vi "RS232_命令(2條直線要寫入雷射的)_VI.vi"(0 "量測值Array(X)":dbl, 1 "量測值Array(Y)":dbl, 2 "功率右":u8=70 max=80, 3 "掃描速率(刀速)右":u16=220 max=2000 format="%0.0f", 5 "error in (no error)":errorcluster, 6 "線段":enum16{"左邊線段", "右邊線段"}(ring), 7 "功率左":u8=70 max=80, 8 "角度(左)":dbl min=0.0 max=360.0, 9 "掃描速率(刀速) 左":u16=220 max=2000 format="%0.0f", 10 "角度(右)":dbl min=0.0 max=360.0, 11 "線段長度左":dbl min=0.0 max=999.0, 13 "線段長度右":dbl) -> (14 "命令字串":string, 19 "error out":errorcluster)   [LabVIEW 2015]
panel:
  out "角度":dbl
  out "X座標":dbl
  out "角度 2":string="-20.000"
  out "X座標 2":string="-20.000"
  out "命令Array":string[](array[string])
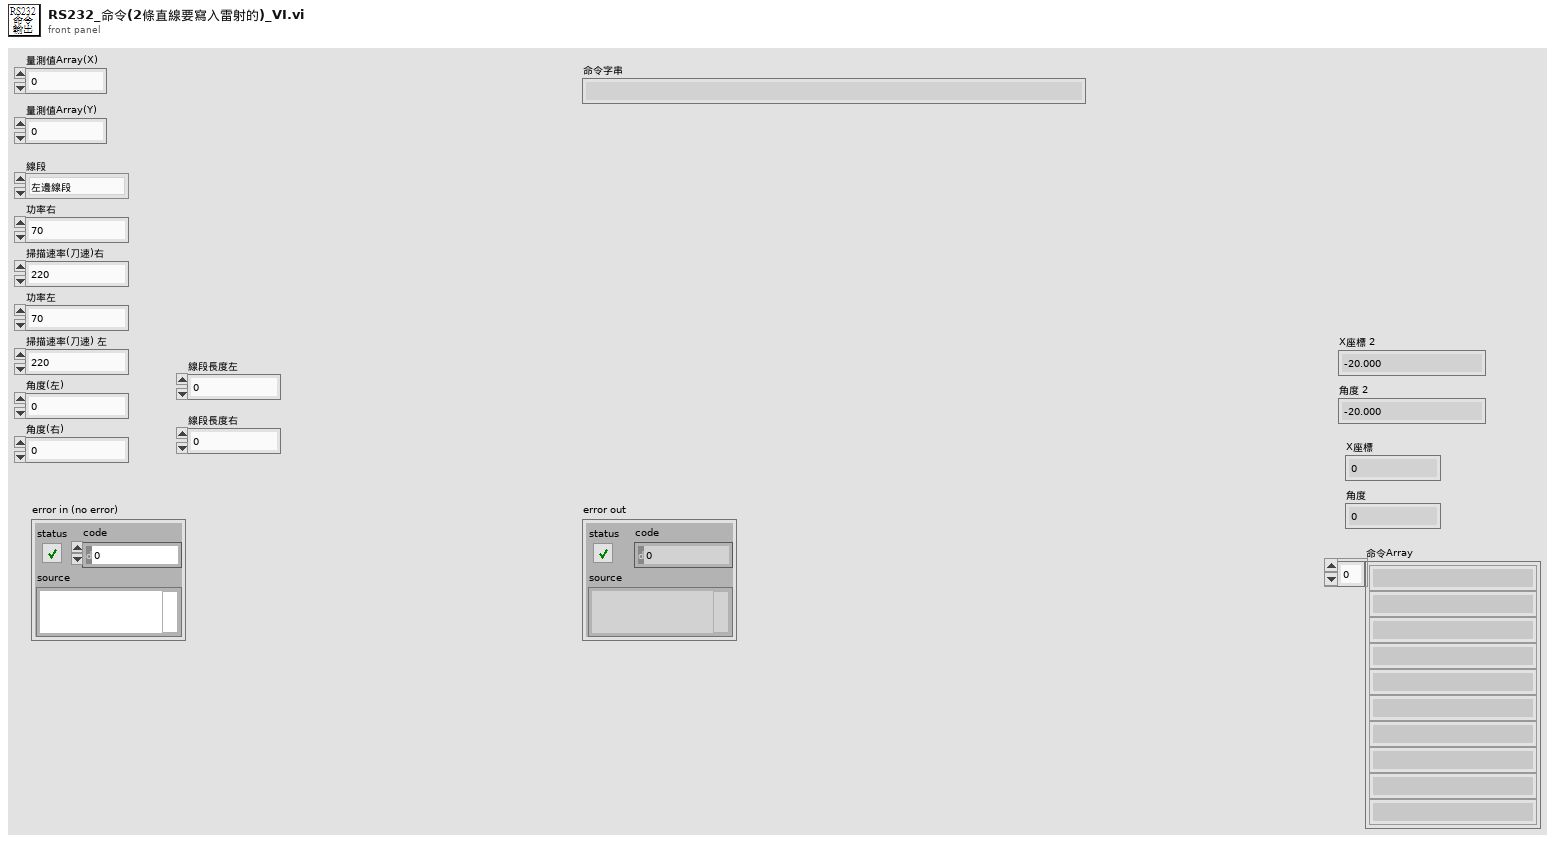
[diagram p1: front panel]
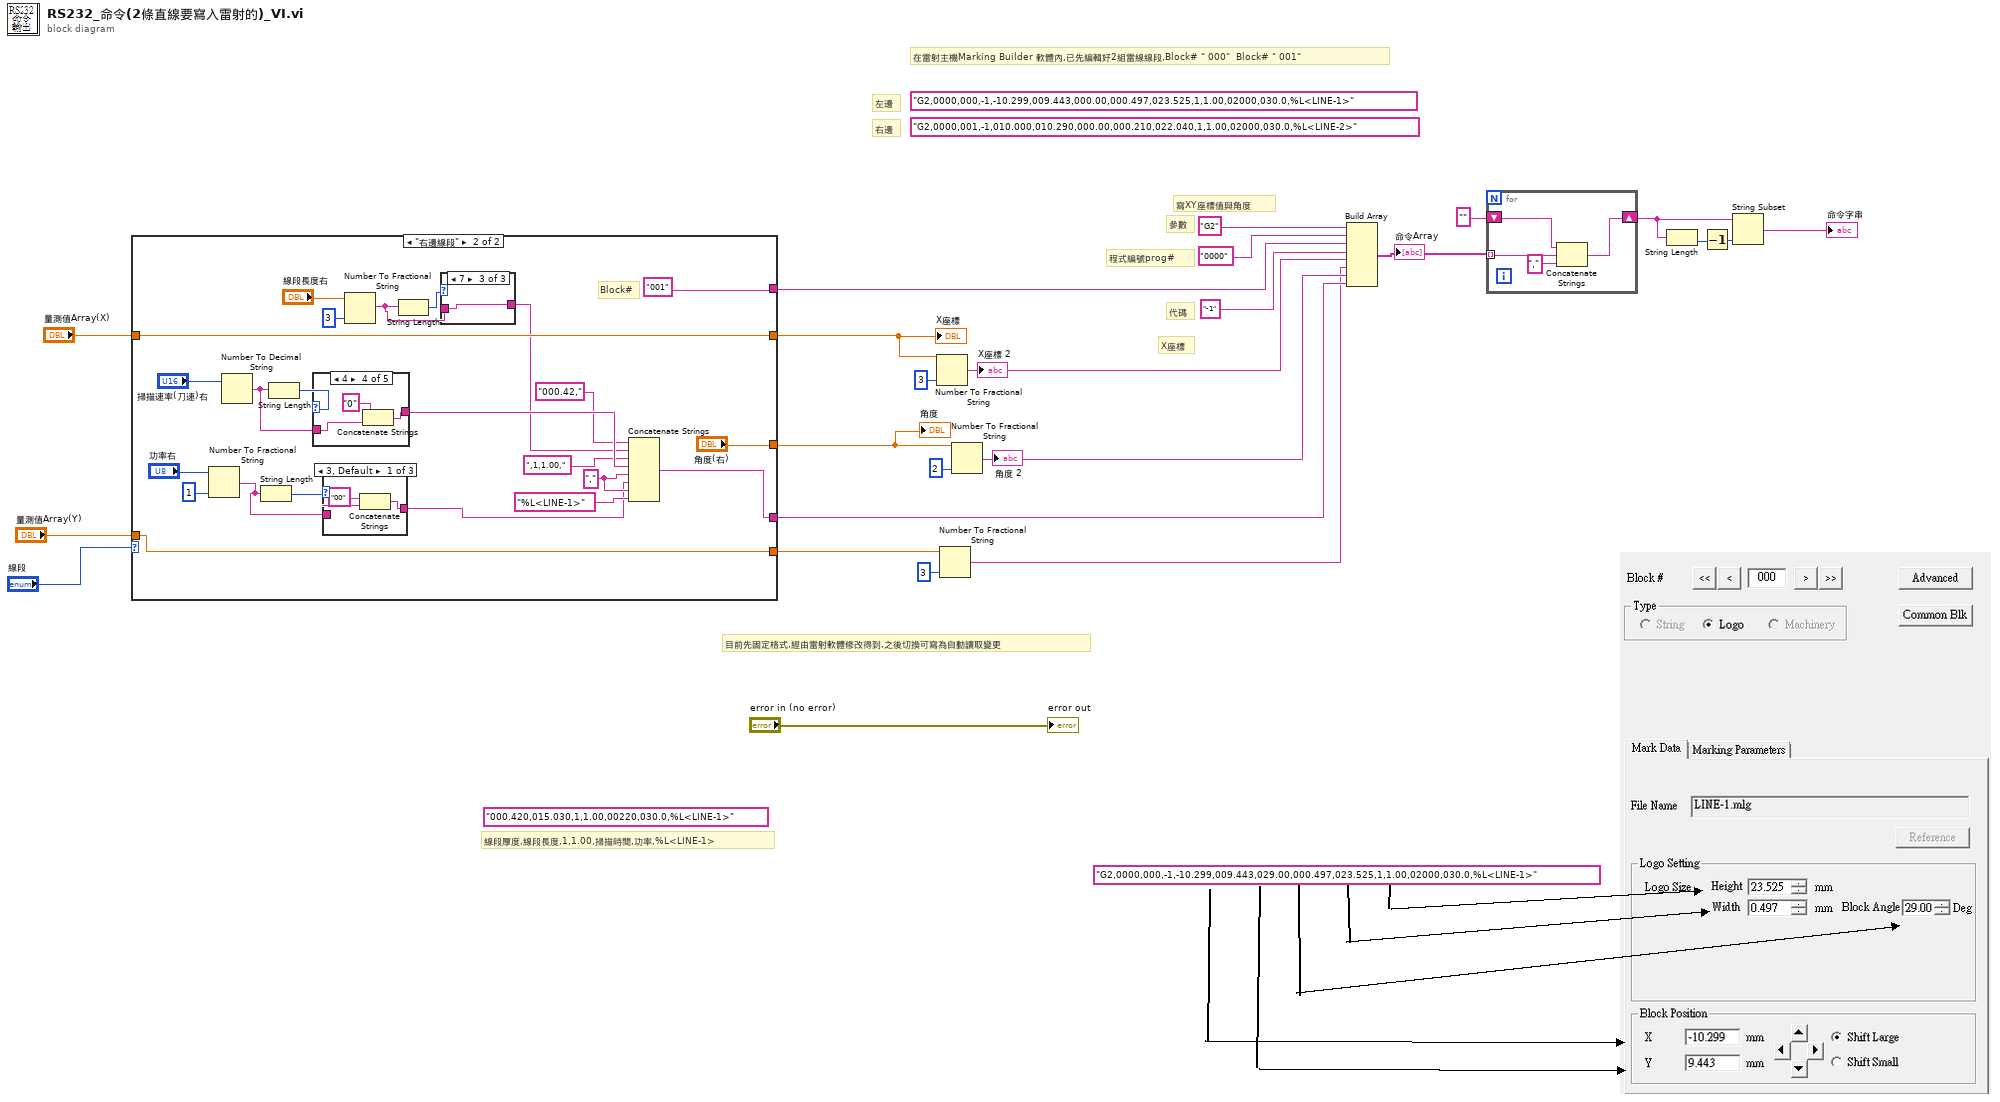
[diagram p0: block diagram]
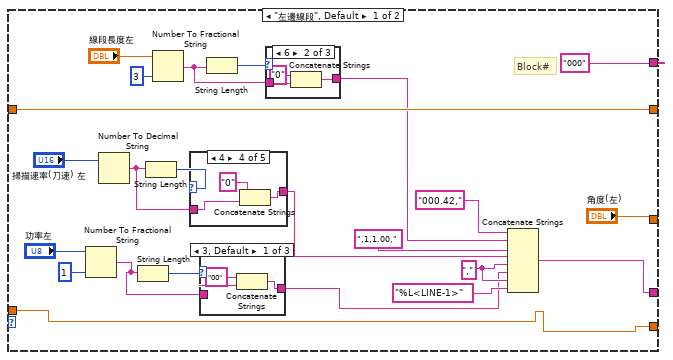
[diagram p2: hidden frame]
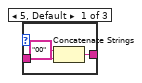
[diagram p3: hidden frame]
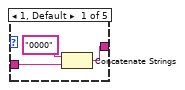
[diagram p5: hidden frame]
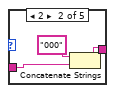
[diagram p6: hidden frame]
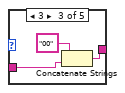
[diagram p7: hidden frame]
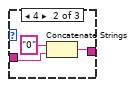
[diagram p9: hidden frame]
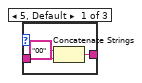
[diagram p11: hidden frame]
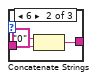
[diagram p12: hidden frame]
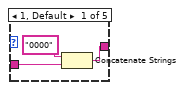
[diagram p13: hidden frame]
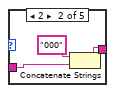
[diagram p14: hidden frame]
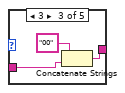
[diagram p15: hidden frame]
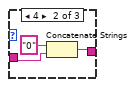
[diagram p17: hidden frame]
diagram:
  (unwired) "000.420,015.030,1,1.00,00220,030.0,%L<LINE-1>"
  (unwired) "G2,0000,000,-1,-10.299,009.443,029.00,000.497,023.525,1,1.00,02000,030.0,%L<LINE-1>"
  (unwired) "G2,0000,001,-1,010.000,010.290,000.00,000.210,022.040,1,1.00,02000,030.0,%L<LINE-2>"
  (unwired) "G2,0000,000,-1,-10.299,009.443,000.00,000.497,023.525,1,1.00,02000,030.0,%L<LINE-1>"
  # "線段厚度,線段長度,1,1.00,掃描時間,功率,%L<LINE-1>"
  # "目前先固定格式,經由雷射軟體修改得到,之後切換可寫為自動讀取變更"
  # "代碼"
  # "右邊"
  # "左邊"
  # "在雷射主機Marking Builder 軟體內,已先編輯好2組雷線線段,Block# \" 000\"  Block# \" 001\""
  # "寫XY座標值與角度"
  # "X座標"
  # "程式編號prog#"
  # "參數"
  n1 = case shown="\"右邊線段\"" "線段" {
    tunnel: [w43 w94] -> w9
    tunnel: ["000" "001"] -> w8
    tunnel: "量測值Array(X)" -> [w32 w83]
    tunnel: [w32 w83] -> w7
    tunnel: ["角度(左)" "角度(右)"] -> w6
    tunnel: "量測值Array(Y)" -> [w31 w82]
    tunnel: [w31 w82] -> w5
    frame "左邊線段", Default {
      w45 = ","
      # "Block#"
      n2 = Number To Fractional String(number="功率左", precision (6)=i16 1 ("width (-)")) -> (F-format string=w38:string)  [unwired: 2 in]
      n3 = Number To Decimal String(number="掃描速率(刀速) 左") -> (decimal integer string=w41:string)  [unwired: 1 in]
      n4 = String Length(string=w38) -> (length=w37:i32)
      n5 = String Length(string=w41) -> (length=w40:i32)
      n6 = Number To Fractional String(number="線段長度左", precision (6)=i16 3) -> (F-format string=w30:string)  [unwired: 2 in]
      n7 = case shown="4" w40 {
        tunnel: w41 -> [w57 w59 w63 w65 w67]
        tunnel: [w55 w58 w61 w64 w67] -> w34
        frame 1, Default {
          n8 = Concatenate Strings("0000" ("string"), w57) -> (w55:string)
        }
        frame 2 {
          n9 = Concatenate Strings("000" ("string"), w59) -> (w58:string)
        }
        frame 3 {
          n10 = Concatenate Strings("00" ("string"), w63) -> (w61:string)
        }
        frame 4 {
          n11 = Concatenate Strings("0" ("string"), w65) -> (w64:string)
        }
        frame 5 {
        }
      }
      n12 = case shown="3, Default" w37 {
        tunnel: w38 -> [w70 w72 w74]
        tunnel: [w68 w71 w74] -> w33
        frame 3, Default {
          n13 = Concatenate Strings("00" ("string"), w70) -> (w68:string)
        }
        frame 4 {
          n14 = Concatenate Strings("0" ("string"), w72) -> (w71:string)
        }
        frame 5 {
        }
      }
      n15 = String Length(string=w30) -> (length=w29:i32)
      n16 = case shown="6" w29 {
        tunnel: w30 -> [w50 w52 w54]
        tunnel: [w48 w53 w54] -> w25
        frame 5, Default {
          n17 = Concatenate Strings("00" ("string"), w50) -> (w48:string)
        }
        frame 6 {
          n18 = Concatenate Strings("0" ("string"), w52) -> (w53:string)
        }
        frame 7 {
        }
      }
      n19 = Concatenate Strings("000.42," ("string"), w25, ",1,1.00,", w34, w45, w33, w45, "%L<LINE-1>" ("string")) -> (w43:string)
    }
    frame "右邊線段" {
      w96 = ","
      # "Block#"
      n20 = Number To Fractional String(number="功率右", precision (6)=i16 1 ("width (-)")) -> (F-format string=w89:string)  [unwired: 2 in]
      n21 = Number To Decimal String(number="掃描速率(刀速)右") -> (decimal integer string=w92:string)  [unwired: 1 in]
      n22 = String Length(string=w89) -> (length=w88:i32)
      n23 = String Length(string=w92) -> (length=w91:i32)
      n24 = case shown="4" w91 {
        tunnel: w92 -> [w107 w109 w113 w115 w117]
        tunnel: [w105 w108 w111 w114 w117] -> w85
        frame 1, Default {
          n25 = Concatenate Strings("0000" ("string"), w107) -> (w105:string)
        }
        frame 2 {
          n26 = Concatenate Strings("000" ("string"), w109) -> (w108:string)
        }
        frame 3 {
          n27 = Concatenate Strings("00" ("string"), w113) -> (w111:string)
        }
        frame 4 {
          n28 = Concatenate Strings("0" ("string"), w115) -> (w114:string)
        }
        frame 5 {
        }
      }
      n29 = case shown="3, Default" w88 {
        tunnel: w89 -> [w120 w122 w124]
        tunnel: [w118 w121 w124] -> w84
        frame 3, Default {
          n30 = Concatenate Strings("00" ("string"), w120) -> (w118:string)
        }
        frame 4 {
          n31 = Concatenate Strings("0" ("string"), w122) -> (w121:string)
        }
        frame 5 {
        }
      }
      n32 = Number To Fractional String(number="線段長度右", precision (6)=i16 3) -> (F-format string=w77:string)  [unwired: 2 in]
      n33 = String Length(string=w77) -> (length=w78:i32)
      n34 = case shown="7" w78 {
        tunnel: w77 -> [w100 w102 w104]
        tunnel: [w98 w103 w104] -> w76
        frame 5, Default {
          n35 = Concatenate Strings("00" ("string"), w100) -> (w98:string)
        }
        frame 6 {
          n36 = Concatenate Strings("0" ("string"), w102) -> (w103:string)
        }
        frame 7 {
        }
      }
      n37 = Concatenate Strings("000.42," ("string"), w76, ",1,1.00,", w85, w96, w84, w96, "%L<LINE-1>" ("string")) -> (w94:string)
    }
  }
  "X座標" <- w7
  "角度" <- w6
  n38 = Number To Fractional String(number=w7, precision (6)=i16 3) -> (F-format string=w13:string)  [unwired: 2 in]
  "X座標 2" <- w13
  n39 = Number To Fractional String(number=w5, precision (6)=i16 3) -> (F-format string=w3:string)  [unwired: 2 in]
  n40 = Number To Fractional String(number=w6, precision (6)=i16 2) -> (F-format string=w11:string)  [unwired: 2 in]
  "角度 2" <- w11
  n41 = Build Array("G2", "0000", w8, "-1", w13, w3, w11, w9) -> (w16:string[])
  "命令Array" <- w16
  n42 = for {
    tunnel: w16 -> [w126] mode=indexing
    shift-right: [w125] -> w21
    shift-left: "" -> [w127]
    n43 = Concatenate Strings(w127, w126, ",") -> (w125:string)
  }
  n44 = String Length(string=w21) -> (length=w22:i32)
  n45 = Decrement(x=w22) -> (x-1=w23:i32)
  n46 = String Subset(string=w21, length (rest)=w23) -> (substring=→"命令字串":string)  [unwired: 1 in]
  "error out" <- "error in (no error)"
